vi "PH_Beamline.color MA-IB BL.vi"(0 "i ref in":refnum<vi>, 2 "Color State MA Input":i32, 5 "error in (no error)":errorcluster) -> (14 "i ref out":refnum<vi>, 19 "error out":errorcluster)   [LabVIEW 2014, in "PH_Beamline.lvlib"]
doc: "This VI colors the MainAmp Injection Box beamline elements."
uses:
  PH_Beamline.lvlib
  PH_StatusHandler/PH_StatusHandler.Status.ctl
  PH_Common/PH_Common.lvlib
  PH_StatusHandler/PH_StatusHandler.lvlib
  PH_BL-Master/PH_BL-Master.lvlib
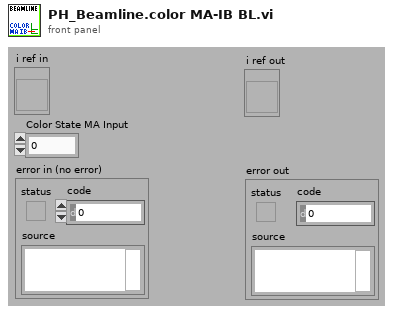
[diagram p1: front panel]
types:
  T1 = typedef "PH_StatusHandler.lvlib/PH_StatusHandler.Status.ctl" = i16
  T2 = typedef "PH_Beamline.lvlib/PH_Beamline.i attribute.ctl" = cluster{"GUI Refs":cluster{"PA ok":refnum<vi>, "MA ok":refnum<vi>, "fs FE ok":refnum<vi>, "ns FE ok":refnum<vi>, "PA ED ok":refnum<vi>, "MAS ok":refnum<vi>, "Booster ok":refnum<vi>, "Mirrortower ok":refnum<vi>, "In.-Box ok":refnum<vi>, "Compressor ok":refnum<vi>, "Experiment LB ok":refnum<vi>, "Experiment LL ok":refnum<vi>, "PHELIX_Beckhoff_Watchdog":refnum<vi>, "Shutters closed":refnum<vi>, "uOPA ok":refnum<vi>, "Vacuum no shotcond Comp LB":refnum<vi>}, "Refs BL MA":refnum<vi>[], "Refs BL MA-IB":refnum<vi>[], "Refs BL fs":refnum<vi>[], "Refs BL PA ED":refnum<vi>[], "Refs BL MAS":refnum<vi>[], "Refs BL Boo":refnum<vi>[], "Refs BL ns":refnum<vi>[], "Refs BL Mirrortower":refnum<vi>[], "Refs BL Compressor":refnum<vi>[], "Refs BL Exp LB":refnum<vi>[], "Radiation Safety":cluster{"Exp Laserbay":cluster{"Ref Op Mode":refnum<vi>, "Ref Laserbay evacuated":refnum<vi>, "Tagname LB evacuated":string, "Shot Mode":T3, "Laserbay evacuated?":i32, "Tagname HV room locked":string, "HV room locked?":i32, "Ref HV room locked":refnum<vi>, "Tagname bridged?":string, "Ref Bridge":refnum<vi>, "I<1E18W/cm²":bool}, "Exp Laserlab":cluster{"Ref Op Mode":refnum<vi>, "Ref Laserlab evacuated":refnum<vi>, "Tagname LL evacuated":string, "Shot Mode":T3, "Laserlab evacuated?":i32, "Tagname bridged?":string, "Ref Bridge":refnum<vi>, "I<1E18W/cm²":bool}}, "Refs BL LL":refnum<vi>[], "PP Igni Heating GUI Refs":refnum<vi>[], "PP Igni Heating Tagnames ":string[], "Refs BL PA":cluster{"undelayed Line before Shutter":refnum<vi>[], "undelayed Line after Shutter":refnum<vi>[], "before Bypass":refnum<vi>[], "delayed Line before Shutter":refnum<vi>[], "delayed Line after Shutter":refnum<vi>[], "before Shutter Input":refnum<vi>[], "after Shutter Input":refnum<vi>[], "Bypass":refnum<vi>[], "before Shutter Exit":refnum<vi>[], "after Shutter Exit":refnum<vi>[], "to MA":refnum<vi>[], "to Lab":refnum<vi>[]}, "BL":cluster{"YLF_BL_Status":i32, "fs_BL_Status":i32, "fs_YLF_BL_Status":i32, "ns_BL_Status":i32, "PA_Input_BL_Status":i32, "PA_UnDelay_BL_Status":i32, "PA_Delay_BL_Status":i32, "PA_BL_Status":i32, "PA_Bypass_BL_Status":i32, "PA_Exit_BL_Status":i32, "PA_LL_BL_Status":i32, "LL_BL_Status":i32, "PA_MA_BL_Status":i32, "MA_Exit_BL_Status":i32, "MA_Z6_BL_Status":i32, "Z6_BL_Status":i32, "MA_LB_BL_Status":i32, "LB_TB2_BL_Status":i32, "PA_before_Bypass_BL_Status":i32, "LB_TB3_BL_Status":i32}, "State Subsystems":cluster{"PA":bool, "MA":bool, "ns FE":bool, "fs FE":bool, "PA ED":bool, "In.-Box":bool, "MAS":bool, "Booster":bool, "Mirrortower":bool, "Compressor":bool, "Experiment LB":bool, "Experiment LL":bool, "uOPA":bool}, "Status Subscriber Information":T4, "Refs BL uOPA":refnum<vi>[], "PA_Input_2_Beam_6PWpGUI not linked?":bool, "PA_Input_Delay_6PGUI not linked?":bool, "Settings":T7}
  T3 = typedef "PH_Beamline.lvlib/PH_Beamline.Operation Mode.ctl" = i32
  T4 = typedef "PH_Beamline.lvlib/PH_Beamline.Status Subscriber Information.ctl" = cluster{"fs Swich YLF":T5, "fs Exit Shutter":T5, "ns Exit Shutter":T5, "PA Input Shutter":T5, "PA PC WP":T5, "PA PC WP 2":T5, "PA Bypass In":T5, "PA Bypass Out":T5, "PA CH 1":T5, "PA delayed":T5, "PA non delayed":T5, "PA Exit Shutter":T5, "PA Switch Lab":T5, "PA Bridge CH Input MA":T5, "MA Diffusor IB":T5, "MA IB Ready":T5, "MA CH 1":T5, "MA CH 2":T5, "MA CH 3":T5, "MA CH 4":T5, "MA Shutter Align Cam":T5, "MA Position MM5":T5, "Calorimeter Switch":T5, "BL Z6 CH 9":T5, "BL Z6 Beamdump":T5, "BL Z6 Shutter":T5, "COS Sensitivity Switch":T5, "Exp LB Shutter":T5, "Exp LB TB 2":T5, "Exp LB TB 3":T5, "PA LL Input CH":T5, "PA LL Output CH":T5, "LL Comp Input Shutter":T5, "LL Comp Output Shutter":T5, "LL Comp FF Shutter":T5, "Exp LL Shutter":T5, "MA IM In IB":T5, "MA IM Out IB":T5, "MA DB In IB":T5, "MA DB Out IB":T5, "Exp LB Shutter Interlock":T5, "Exp LL Shutter Interlock":T5, "MM1 Force Sensor":T5}
  T5 = typedef "PH_BL-Master.lvlib/PH_BL-Master.Status Subscriber Information.ctl" = cluster{"Index of element":i32, "Attributeset":T6}
  T6 = typedef "PH_BL-Master.lvlib/PH_BL-Master.Attribute Set.ctl" = enum16{"Boolean Status Service Subscriber", "Picture Status Service Subscriber"}
  T7 = typedef "PH_Beamline_Chief.lvlib/PH_Beamline_Chief.Settings.ctl" = cluster{"PA Doublepass Mode":bool, "Compressor Vaccuum LB not relevant":bool, "Windowshutter TB2 not relevant":bool, "Windowshutter TB3 not relevant":bool}
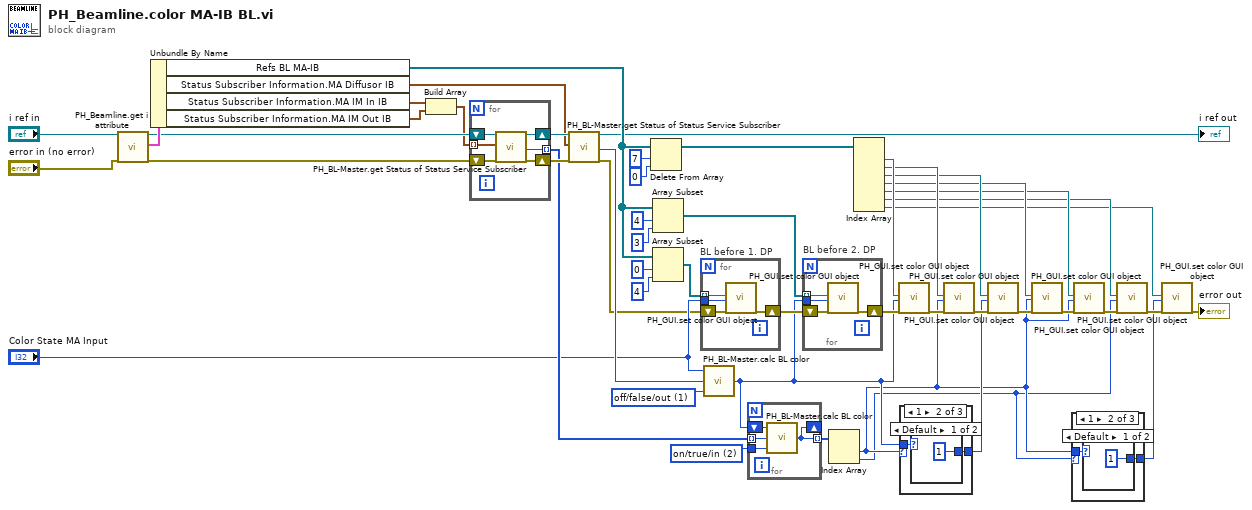
[diagram p0: block diagram]
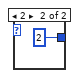
[diagram p3: hidden frame]
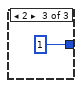
[diagram p4: hidden frame]
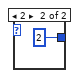
[diagram p6: hidden frame]
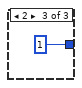
[diagram p7: hidden frame]
diagram:
  w19 = T1 2 items=["no info", "off/false/out", "on/true/in", "Failure", "Alarm", "Status 1", "Status 2", "Status 3"] ("State for \"2\" (on) of ABLE (off/false/out)")
  w18 = T1 1 items=["no info", "off/false/out", "on/true/in", "Failure", "Alarm", "Status 1", "Status 2", "Status 3"] ("State for \"2\" (on) of ABLE (off/false/out)")
  n1 = call "PH_Beamline.get i attribute.vi"("i ref in"="i ref in", "error in (no error)"="error in (no error)") -> ("i ref out"=w7:refnum<vi>, "i attribute"=w45:T2, "error out"=w5:errorcluster)  [unwired: 15 in]
  n2 = Unbundle By Name(w45) -> ("Refs BL MA-IB"=w43:refnum<vi>[], "Status Subscriber Information.MA Diffusor IB"=w4:T5, "Status Subscriber Information.MA IM In IB"=w3:T5, "Status Subscriber Information.MA IM Out IB"=w2:T5)
  n3 = Build Array(w3, w2) -> (w1:T5[])
  n4 = for {
    tunnel: w1 -> [w55] mode=indexing
    tunnel: [w52] -> w21 mode=indexing
    shift-right: [w54] -> w24
    shift-left: w7 -> [w51]
    shift-right: [w53] -> w23
    shift-left: w5 -> [w56]
    n5 = call "PH_BL-Master.get Status of Status Service Subscriber.vi"("i ref in"=w51, "Wanted Status Subscriber Information"=w55, "error in (no error)"=w56) -> ("i ref out"=w54:refnum<vi>, "Status"=w52:T1, "error out"=w53:errorcluster)  [unwired: 11 in, 3 out]
  }
  n6 = call "PH_BL-Master.get Status of Status Service Subscriber.vi"("i ref in"=w24, "Wanted Status Subscriber Information"=w4, "error in (no error)"=w23) -> ("i ref out"=→"i ref out":refnum<vi>, "Status"=w22:T1, "error out"=w9:errorcluster)  [unwired: 11 in, 3 out]
  n7 = Delete From Array(array=w43, length=7, index=0) -> (array with subset deleted=w40:refnum<vi>[])  [unwired: 1 out]
  n8 = Array Subset(array=w43, index=4, length=3) -> (w46:refnum<vi>[])
  n9 = Array Subset(array=w43, index=0, length=4) -> (w17:refnum<vi>[])
  n10 = for "BL before 1. DP" {
    tunnel: w17 -> [w60] mode=indexing
    shift-right: [w58] -> w47
    shift-left: w9 -> [w59]
    tunnel: "Color State MA Input" -> [w57]
    n11 = call "PH_GUI.set color GUI object.vi"("GUI object Ref"=w60, "State"=w57, "error in (no error)"=w59) -> ("error out"=w58:errorcluster)  [unwired: 16 in]
  }
  n12 = call "PH_BL-Master.calc BL color.vi"("State for \"2\" (on) of ABLE (off/false/out)"=w18, "State ABLE"=w22, "State before ABLE"="Color State MA Input") -> ("State after ABLE"=w15:i32)
  n13 = for {
    tunnel: w21 -> [w61] mode=indexing
    tunnel: [w62] -> w20 mode=indexing
    tunnel: w19 -> [w63]
    shift-right: [w62] -> _
    shift-left: w15 -> [w64]
    n14 = call "PH_BL-Master.calc BL color.vi"("State for \"2\" (on) of ABLE (off/false/out)"=w63, "State ABLE"=w61, "State before ABLE"=w64) -> ("State after ABLE"=w62:i32)
  }
  n15 = for "BL before 2. DP" {
    tunnel: w46 -> [w68] mode=indexing
    shift-right: [w66] -> w39
    shift-left: w47 -> [w67]
    tunnel: w15 -> [w65]
    n16 = call "PH_GUI.set color GUI object.vi"("GUI object Ref"=w68, "State"=w65, "error in (no error)"=w67) -> ("error out"=w66:errorcluster)  [unwired: 16 in]
  }
  n17 = Index Array(array=w20) -> (element #1=w12:i32, element #2=w11:i32)  [unwired: 2 in]
  n18 = Index Array(array=w40) -> (element #1=w38:refnum<vi>, element #2=w37:refnum<vi>, element #3=w36:refnum<vi>, element #4=w35:refnum<vi>, element #5=w34:refnum<vi>, element #6=w29:refnum<vi>, element #7=w28:refnum<vi>)  [unwired: 7 in]
  n19 = call "PH_GUI.set color GUI object.vi"("GUI object Ref"=w38, "State"=w15, "error in (no error)"=w39) -> ("error out"=w26:errorcluster)  [unwired: 16 in]
  n20 = case shown="1" w12 {
    selector: w12 -> [w69 _ _]
    tunnel: [w69 w71 1 ("State after ABLE")] -> w13
    tunnel: w15 -> [_ w70 _]
    frame Default {
    }
    frame 1 {
      n21 = case shown="Default" w70 {
        tunnel: [1 ("State after ABLE") 2 ("State after ABLE")] -> w71
        frame Default {
        }
        frame 2 {
        }
      }
    }
    frame 2 {
    }
  }
  n22 = call "PH_GUI.set color GUI object.vi"("GUI object Ref"=w37, "State"=w12, "error in (no error)"=w26) -> ("error out"=w33:errorcluster)  [unwired: 16 in]
  n23 = call "PH_GUI.set color GUI object.vi"("GUI object Ref"=w36, "State"=w13, "error in (no error)"=w33) -> ("error out"=w32:errorcluster)  [unwired: 16 in]
  n24 = call "PH_GUI.set color GUI object.vi"("GUI object Ref"=w35, "State"=w12, "error in (no error)"=w32) -> ("error out"=w31:errorcluster)  [unwired: 16 in]
  n25 = case shown="1" w11 {
    selector: w11 -> [w75 _ _]
    tunnel: [w75 w77 1 ("State after ABLE")] -> w14
    tunnel: w12 -> [_ w76 _]
    frame Default {
    }
    frame 1 {
      n26 = case shown="Default" w76 {
        tunnel: [1 ("State after ABLE") 2 ("State after ABLE")] -> w77
        frame Default {
        }
        frame 2 {
        }
      }
    }
    frame 2 {
    }
  }
  n27 = call "PH_GUI.set color GUI object.vi"("GUI object Ref"=w34, "State"=w12, "error in (no error)"=w31) -> ("error out"=w30:errorcluster)  [unwired: 16 in]
  n28 = call "PH_GUI.set color GUI object.vi"("GUI object Ref"=w29, "State"=w11, "error in (no error)"=w30) -> ("error out"=w27:errorcluster)  [unwired: 16 in]
  n29 = call "PH_GUI.set color GUI object.vi"("GUI object Ref"=w28, "State"=w14, "error in (no error)"=w27) -> ("error out"=→"error out":errorcluster)  [unwired: 16 in]
